vi "DS3231_Decode_Time_Datavi.vi"(11 "Raw_RTC_Data_In":u8[](array[numeric]) format="%2x") -> (3 "DS3231_Date_Time":T1)   [LabVIEW 2022 SP3]
doc: "Petrus Prins\n31 July 2026"
uses:
  DS3231_Date_Time.ctl
  <vilib>/MakerHub/Toolbox/LMH-Toolbox.lvlib
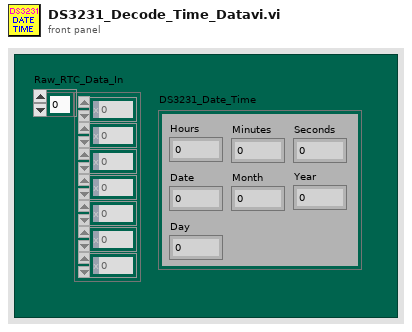
[diagram p1: front panel]
types:
  T1 = typedef "DS3231_Date_Time.ctl" = cluster{"Seconds":u16, "Minutes":u16, "Hours":u16, "Day":u16, "Date":u16, "Month":u16, "Year":u16}
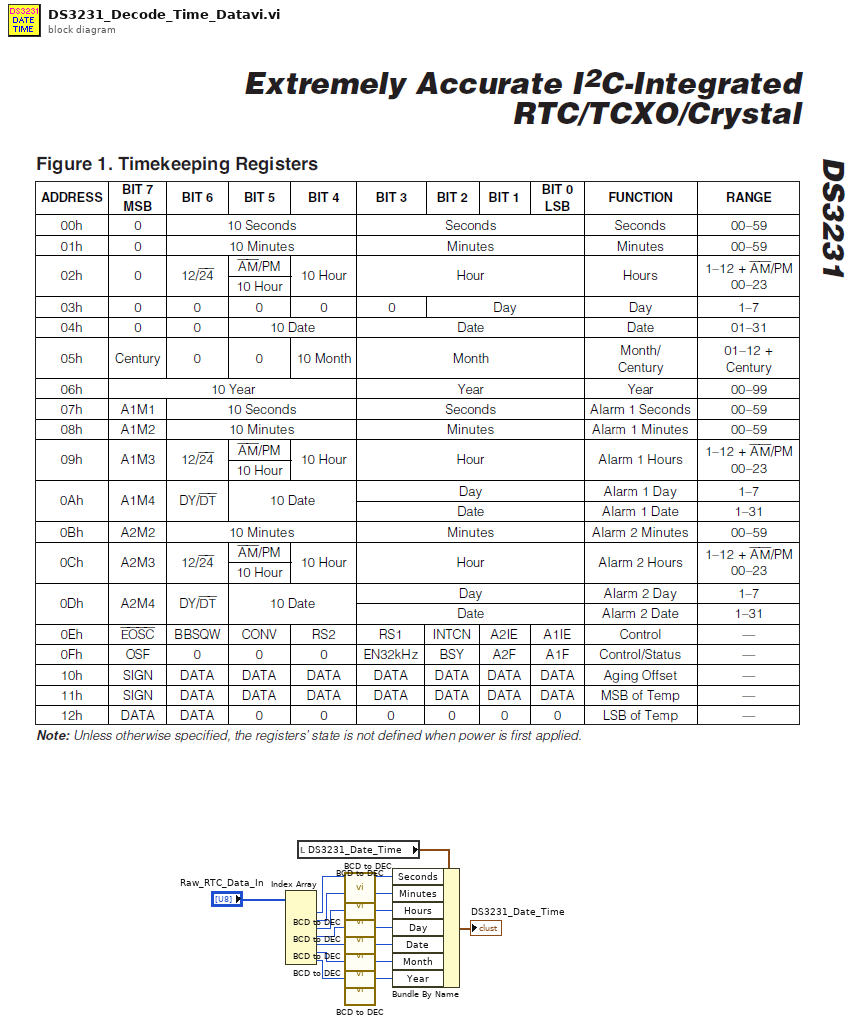
[diagram p0: block diagram]
diagram:
  n1 = Index Array(array="Raw_RTC_Data_In") -> (element #1=w17:u8, element #2=w16:u8, element #3=w15:u8, element #4=w14:u8, element #5=w13:u8, element #6=w12:u8, element #7=w11:u8)  [unwired: 7 in]
  n2 = local read "DS3231_Date_Time"() -> (w9:T1)
  n3 = call <vilib>:"BCD to DEC.vi"("BCD"=w17) -> ("DEC"=w8:u16)  [unwired: 10 in]
  n4 = call <vilib>:"BCD to DEC.vi"("BCD"=w16) -> ("DEC"=w7:u16)  [unwired: 10 in]
  n5 = call <vilib>:"BCD to DEC.vi"("BCD"=w15) -> ("DEC"=w6:u16)  [unwired: 10 in]
  n6 = call <vilib>:"BCD to DEC.vi"("BCD"=w14) -> ("DEC"=w5:u16)  [unwired: 10 in]
  n7 = call <vilib>:"BCD to DEC.vi"("BCD"=w13) -> ("DEC"=w4:u16)  [unwired: 10 in]
  n8 = call <vilib>:"BCD to DEC.vi"("BCD"=w12) -> ("DEC"=w3:u16)  [unwired: 10 in]
  n9 = call <vilib>:"BCD to DEC.vi"("BCD"=w11) -> ("DEC"=w2:u16)  [unwired: 10 in]
  n10 = Bundle By Name(cluster=w9, "Seconds"=w8, "Minutes"=w7, "Hours"=w6, "Day"=w5, "Date"=w4, "Month"=w3, "Year"=w2) -> (→"DS3231_Date_Time":T1)
